vi "Hoorizontal coords to select indent Wrapper.vi"(4 "DragStart.Drag Indices":i32[](array[numeric]), 6 "DragStart.DragOver Same?":bool, 7 "Displayed Row":i32, 8 "Coords.Horizontal":i32, 9 "Tree.Position:Left":i32, 10 "TreeItem Indices (Displayed Items)":i32[](array[numeric]), 11 "TreeItems":T2[](array[typedef])) -> (0 "Bar type":T1=enum."tilda up", 1 "Allowed?":bool, 2 "indent":i32, 3 "Insertion index":i32)   [LabVIEW 2020, in "BetterDragAndDrop.lvlib" / "BetterTreeHandle.lvclass"]
uses:
  Classes/BetterTreeHandle/BetterTreeHandle.lvclass
  Classes/BetterTreeItem/SubVIs/TreeItem.ctl
  Classes/BetterTreeBar/SubVIs/Horizontal Bar Enumeration.ctl
  Classes/BetterTreeBar/BetterHorizontalBar.lvclass
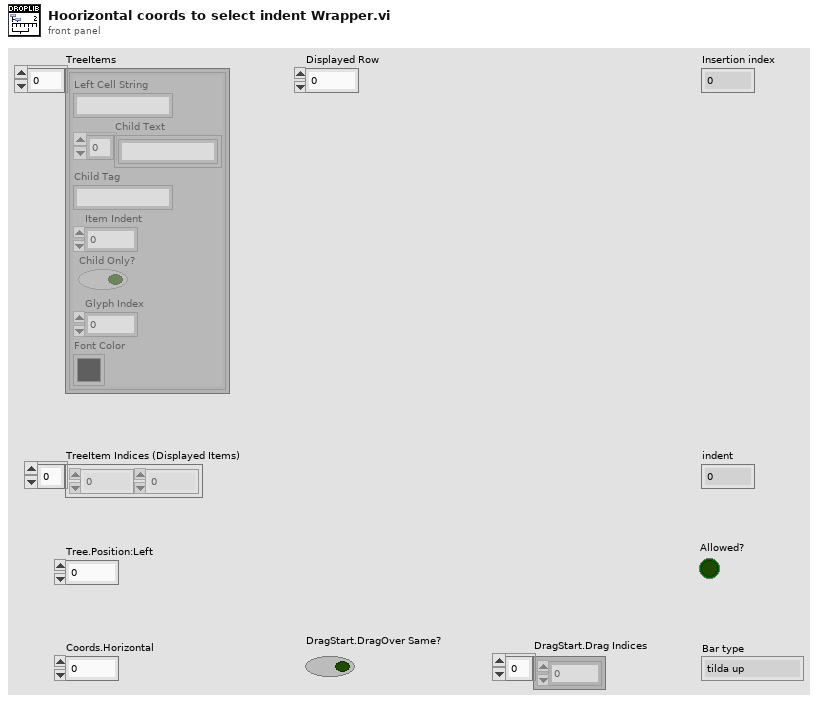
[diagram p1: front panel]
types:
  T1 = typedef "BetterDragAndDrop.lvlib/BetterHorizontalBar.lvclass/Horizontal Bar Enumeration.ctl" = enum16{"None", "only bar", "tilda up"}
  T2 = typedef "BetterDragAndDrop.lvlib/BetterTreeHandle.lvclass/TreeItem.ctl" = cluster{"Left Cell String":string, "Child Text":string[], "Child Tag":string, "Item Indent":i32, "Child Only?":bool, "Glyph Index":i32, "Font Color":u32}
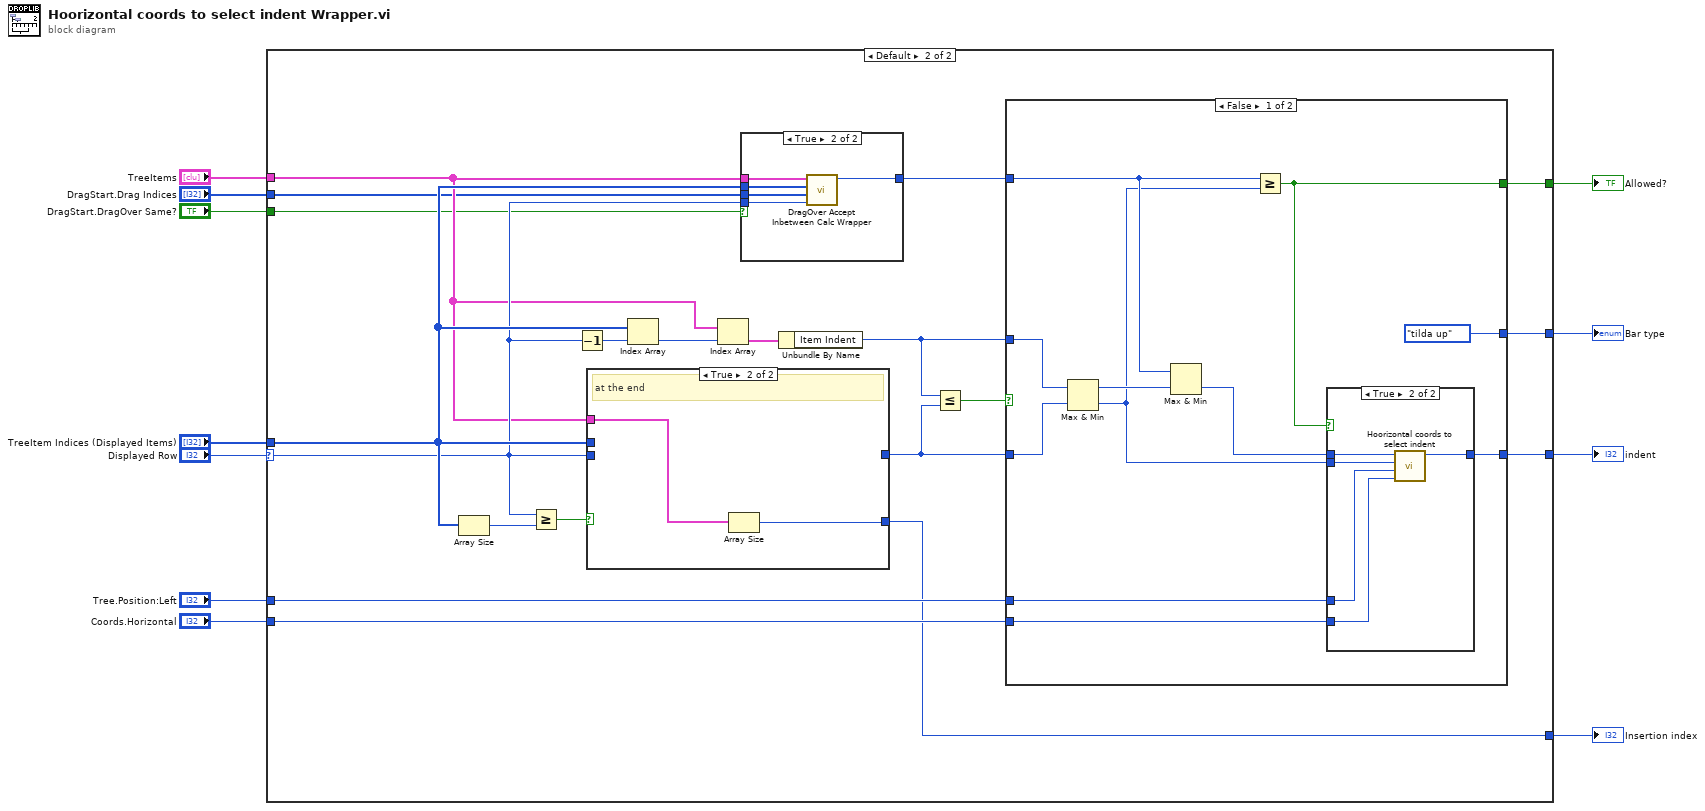
[diagram p0: block diagram]
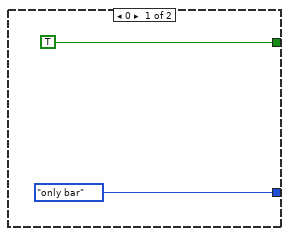
[diagram p2: hidden frame]
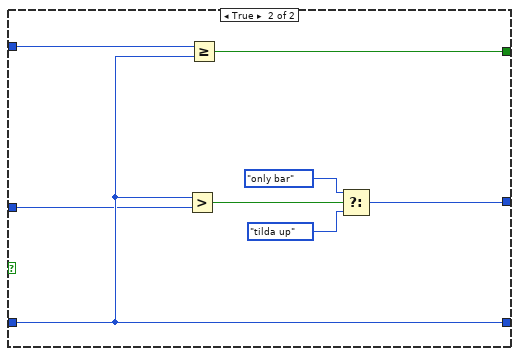
[diagram p4: hidden frame]
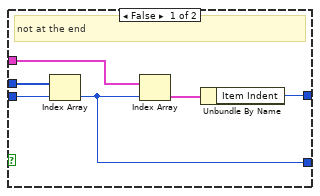
[diagram p5: hidden frame]
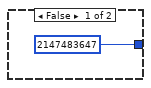
[diagram p6: hidden frame]
diagram:
  n1 = case shown="Default" "Displayed Row" {
    selector: "Displayed Row" -> [_ w22]
    tunnel: "TreeItem Indices (Displayed Items)" -> [_ w23]
    tunnel: "TreeItems" -> [_ w19]
    tunnel: "Tree.Position:Left" -> [_ w31]
    tunnel: "Coords.Horizontal" -> [_ w30]
    tunnel: [_ w29] -> w6
    tunnel: [TRUE w26] -> w5
    tunnel: [_ w21] -> w4
    tunnel: [Horizontal_Bar_Enumeration."only bar" ("New Value") w16] -> w3
    tunnel: "DragStart.Drag Indices" -> [_ w15]
    tunnel: "DragStart.DragOver Same?" -> [_ w14]
    frame 0 {
    }
    frame Default {
      n2 = Array Size(array=w23) -> (size(s)=w24:i32)
      n3 = Greater Or Equal?(x=w22, y=w24) -> (x >= y?=w20:bool)
      n4 = Decrement(x=w22) -> (x-1=w33:i32)
      n5 = case shown="True" w20 {
        tunnel: w19 -> [w64 w66]
        tunnel: [w62 _] -> w18
        tunnel: w23 -> [w61 _]
        tunnel: w22 -> [w60 _]
        tunnel: [w59 w65] -> w21
        frame False {
          # "not at the end"
          n6 = Index Array(array=w61, index=w60) -> (element=w59:i32)
          n7 = Index Array(array=w64, index=w59) -> (element=w63:T2)
          n8 = Unbundle By Name(w63) -> ("Item Indent"=w62:i32)
        }
        frame True {
          # "at the end"
          n9 = Array Size(array=w66) -> (size(s)=w65:i32)
        }
      }
      n10 = Index Array(array=w23, index=w33) -> (element=w32:i32)
      n11 = Index Array(array=w19, index=w32) -> (element=w28:T2)
      n12 = case shown="True" w14 {
        tunnel: w15 -> [_ w72]
        tunnel: w23 -> [_ w71]
        tunnel: w22 -> [_ w70]
        tunnel: w19 -> [_ w69]
        tunnel: [2147483647 ("max indent allowed") w68] -> w25
        frame False {
        }
        frame True {
          n13 = call "DragOver Accept Inbetween Calc Wrapper.vi"("Displayed Row"=w70, "TreeItem Indices (DragStart)"=w72, "TreeItem Indices (Displayed Items)"=w71, "TreeItems"=w69) -> ("max indent allowed"=w68:i32)  [unwired: 7 in]
        }
      }
      n14 = Unbundle By Name(w28) -> ("Item Indent"=w17:i32)
      n15 = Less Or Equal?(x=w17, y=w18) -> (x <= y?=w27:bool)
      n16 = case shown="False" w27 {
        tunnel: [w44 w56] -> w29
        tunnel: w30 -> [w43 _]
        tunnel: w31 -> [w42 _]
        tunnel: w18 -> [w39 w56]
        tunnel: w25 -> [w37 w58]
        tunnel: [w35 w57] -> w26
        tunnel: w17 -> [w40 w55]
        tunnel: [Horizontal_Bar_Enumeration."tilda up" ("New Value") w51] -> w16
        frame False {
          n17 = Max & Min(x=w40, y=w39) -> (max(x,y)=w41:i32, min(x,y)=w36:i32)
          n18 = Max & Min(x=w37, y=w41) -> (min(x,y)=w38:i32)  [unwired: 1 out]
          n19 = Greater Or Equal?(x=w37, y=w36) -> (x >= y?=w35:bool)
          n20 = case shown="True" w35 {
            tunnel: [w45 w50] -> w44
            tunnel: w43 -> [_ w49]
            tunnel: w42 -> [_ w48]
            tunnel: w38 -> [_ w47]
            tunnel: w36 -> [w45 w46]
            frame False {
            }
            frame True {
              n21 = call "Hoorizontal coords to select indent.vi"("Coords.Horizontal"=w49, "Tree.Position:Left"=w48, "min allowed indent"=w46, "max allowed indent"=w47) -> ("Coord Selected indent"=w50:i32)  [unwired: 7 in]
            }
          }
        }
        frame True {
          n22 = Greater?(x=w56, y=w55) -> (0:w54:bool)
          n23 = Greater Or Equal?(x=w58, y=w56) -> (x >= y?=w57:bool)
          n24 = Select(t=Horizontal_Bar_Enumeration."only bar" ("New Value"), s=w54, f=Horizontal_Bar_Enumeration."tilda up" ("New Value")) -> (s? t:f=w51:T1)
        }
      }
    }
  }
  "indent" <- w6
  "Allowed?" <- w5
  "Insertion index" <- w4
  "Bar type" <- w3
